vi "氨氮总磷质控流程.vi"(9 "总磷1":bool, 10 "氨氮1":bool, 11 "队列输入":refnum<queue>) -> (3 "布尔":bool)   [LabVIEW 2016, in "质控单元.lvlib"]
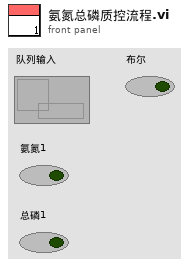
[diagram p1: front panel]
types:
  T1 = enum16{"待机", "启动氨氮水样", "氨氮测量中", "启动氨氮加标", "启动氨氮加标回收", "氨氮加标回收测量中", "启动总磷水样", "总磷水样测量中", "启动总磷加标", "启动总磷加标回收", "总磷加标回收测量中", "结束"}
  T2 = cluster{"站号":u16, "量程切换":enum32{"H", "L", "AUTO"}, "控制命令":enum16{"启动测量", "标样核查", "零点核查", "跨度核查", "空白测试", "平行样测试", "加标回收", "空白校准", "标样校准", "初始化（清洗）", "停止测试", "仪器重启", "校时", "模式设置", "测量间隔设置", "盲样测试"}, "模式设置":enum16{"待机", "连续模式", "周期模式", "定点模式", "受控模式", "手动模式"}, "测量间隔":u16}
  T3 = cluster{"时间标识":timestamp, "设备":string, "日志信息":string}
  T4 = cluster{"系统时间":timestamp, "工作状态":enum16{"空闲", "水样测试", "标样核查", "零点核查", "跨度核查", "空白测试", "平行样测试", "加标回收", "空白校准", "标样校准", "初始化（清洗）"}, "测量模式":enum16{"待机", "连续模式", "周期模式", "定点模式", "受控模式", "手动模式"}, "告警代码":enum16{"无告警", "缺试剂告警", "缺水样告警", "缺蒸馏水告警", "缺标液告警", "仪表漏液告警", "标定异常告警", "超量程告警", "加热异常", "低试剂预警", "超上限告警", "超下限告警", "仪表内部其他异常", "滴定异常告警", "电极异常告警", "量程切换告警", "参数设置告警", "PH电极电位异常", "电导率电极异常", "浊度光度异常", "溶解氧电极异常", "溶解氧光强异常", "温度异常告警", "PH异常告警", "溶解氧异常告警", "电导率异常告警", "浊度异常告警", "叶绿素异常告警", "藻密度异常告警", "蓝绿藻异常告警", "ORP异常告警", "氨氮异常告警", "清洁刷异常告警", "SD卡异常告警", "蓝牙异常告警", "Wifi异常告警", "流程异常告警"}, "故障代码":enum16{"无故障", "电机故障", "温度故障", "通讯故障", "滴定故障"}, "日志代码":u16, "软件版本":u16, "F0":sgl, "F1":sgl, "F2":sgl, "F3":sgl, "T":sgl, "H":sgl, "id":u16, "flowid":u16, "量程":u16}
  T5 = enum16{"空闲", "水样测试", "标样核查", "零点核查", "跨度核查", "空白测试", "平行样测试", "加标回收", "空白校准", "标样校准", "初始化（清洗）"}
  T6 = cluster{"因子编码":u32, "单位":u16, "标样参考值":sgl, "水样数据时间":timestamp, "水样实测值":sgl, "水样数据标识":string, "标样数据时间":timestamp, "标样实测值":sgl, "标样数据标识":string, "空白数据时间":timestamp, "空白实测值":sgl, "空白数据标识":string, "零点核查数据时间":timestamp, "零点核查实测值":sgl, "零点核查数据标识":string, "跨度核查数据时间":timestamp, "跨度核查实测值":sgl, "跨度核查数据标识":string, "加标回收数据时间":timestamp, "加标回收实测值":sgl, "加标回收数据标识":string, "平行样数据时间":timestamp, "平行样实测值":sgl, "平行样数据标识":string}
  T7 = cluster{"量程":dbl, "检出限":dbl, "加标前水样浓度":dbl, "加标后水样浓度":dbl, "加标水杯定容体积":dbl, "加标母液浓度":dbl, "加标体积":dbl, "加标回收率":dbl}
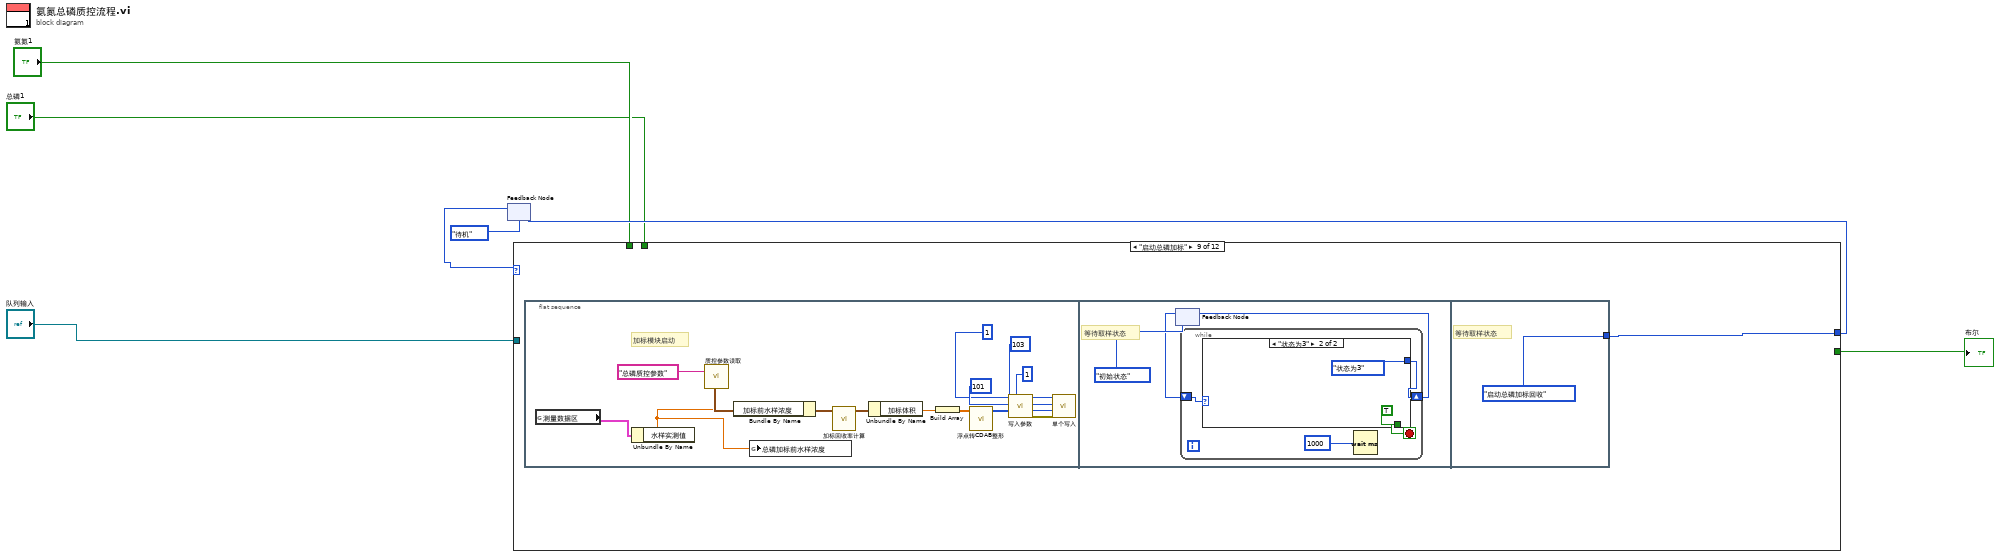
[diagram p0: block diagram]
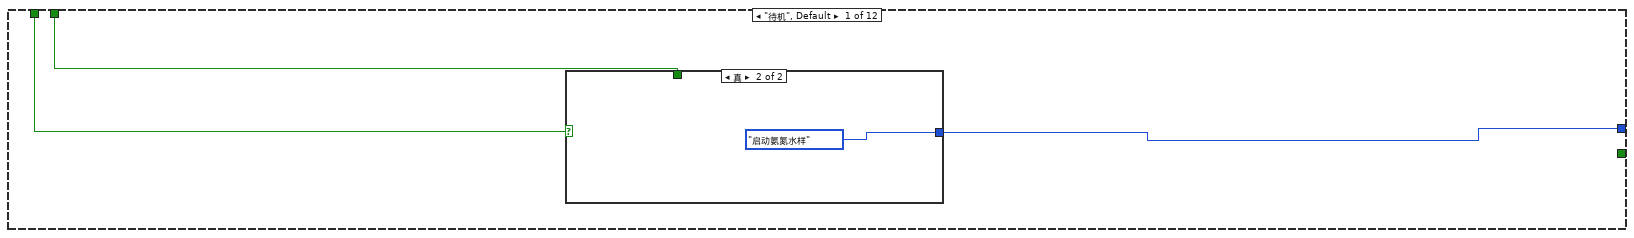
[diagram p2: hidden frame]
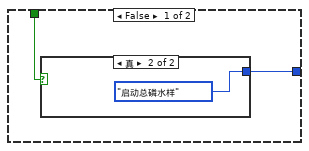
[diagram p3: hidden frame]
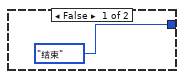
[diagram p4: hidden frame]
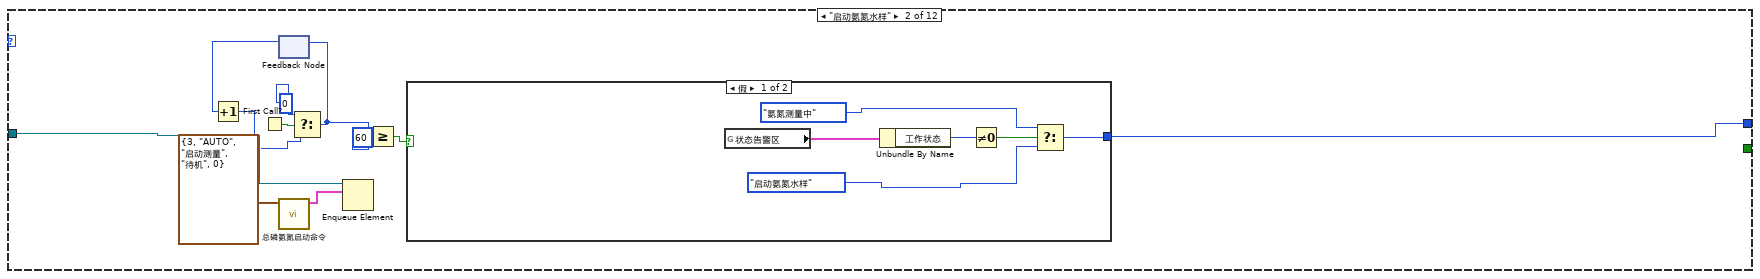
[diagram p5: hidden frame]
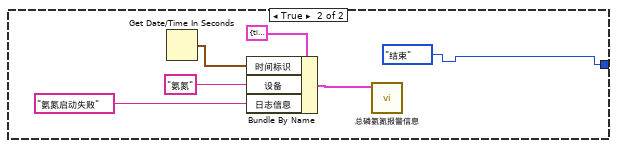
[diagram p6: hidden frame]
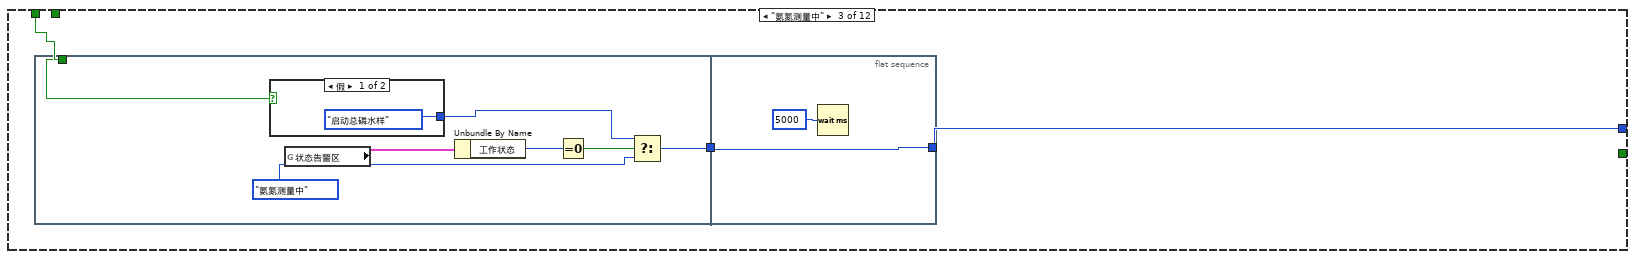
[diagram p7: hidden frame]
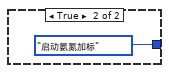
[diagram p8: hidden frame]
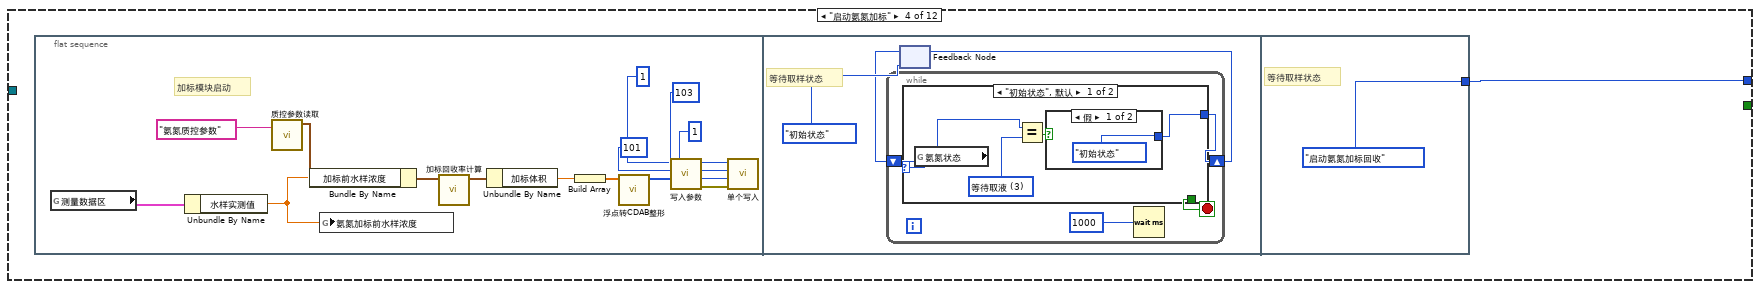
[diagram p9: hidden frame]
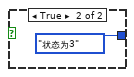
[diagram p10: hidden frame]
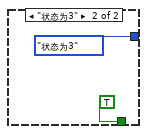
[diagram p11: hidden frame]
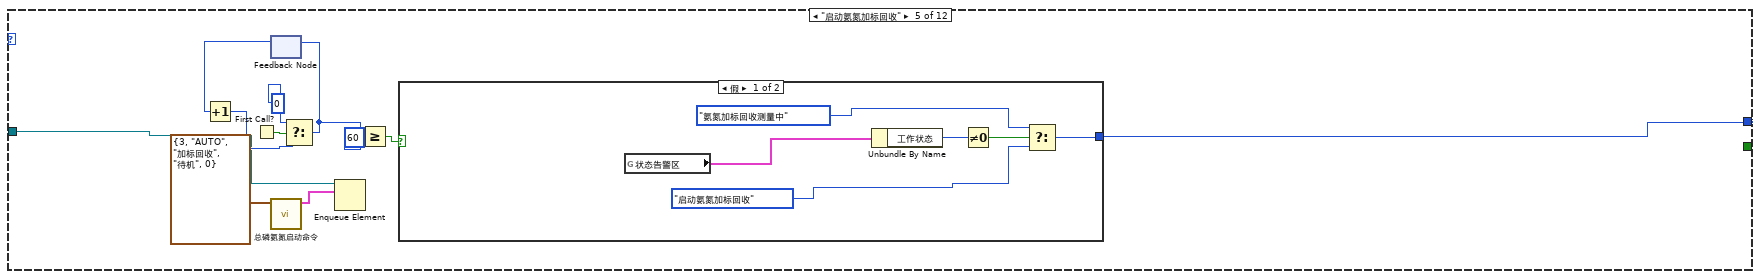
[diagram p12: hidden frame]
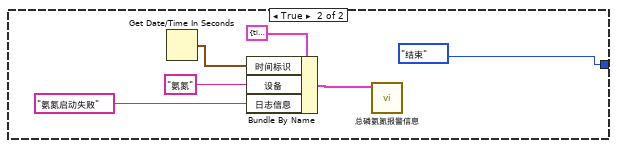
[diagram p13: hidden frame]
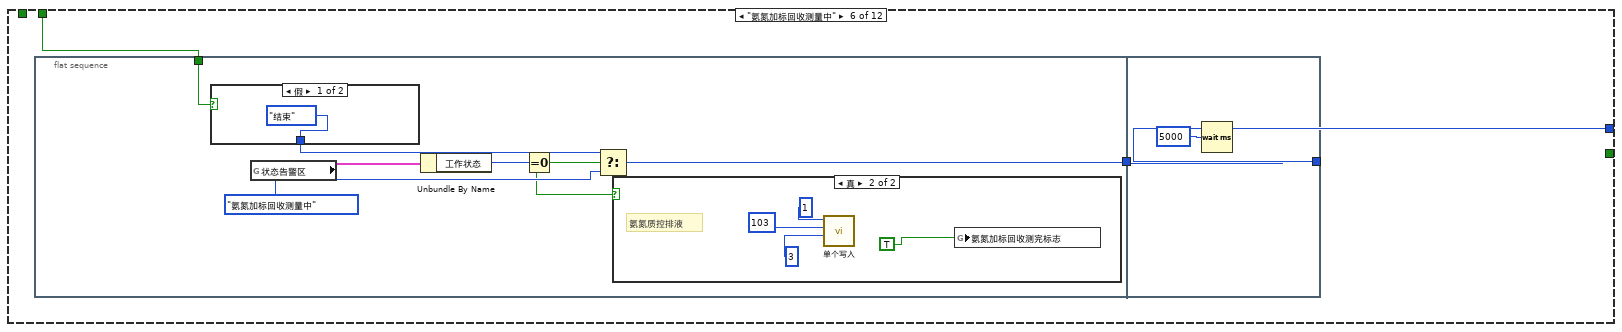
[diagram p14: hidden frame]
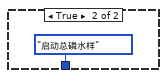
[diagram p15: hidden frame]
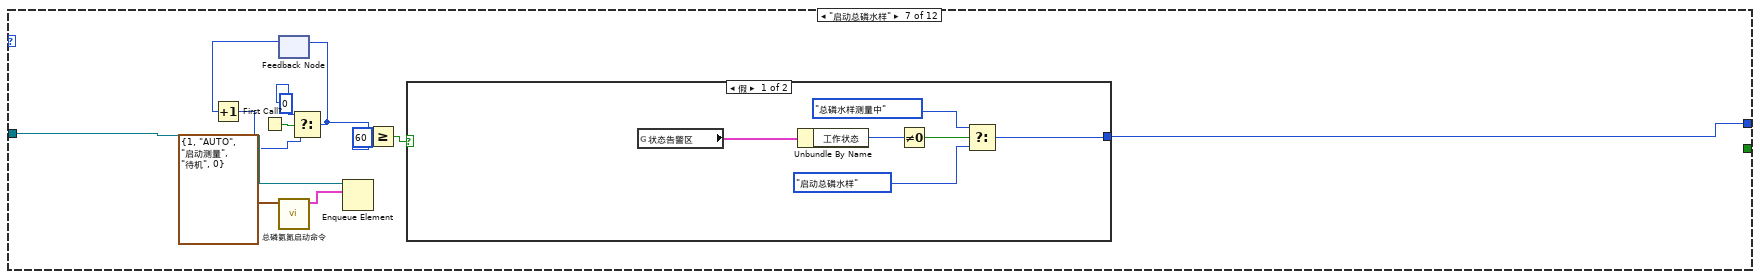
[diagram p17: hidden frame]
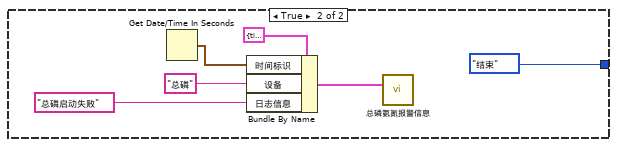
[diagram p18: hidden frame]
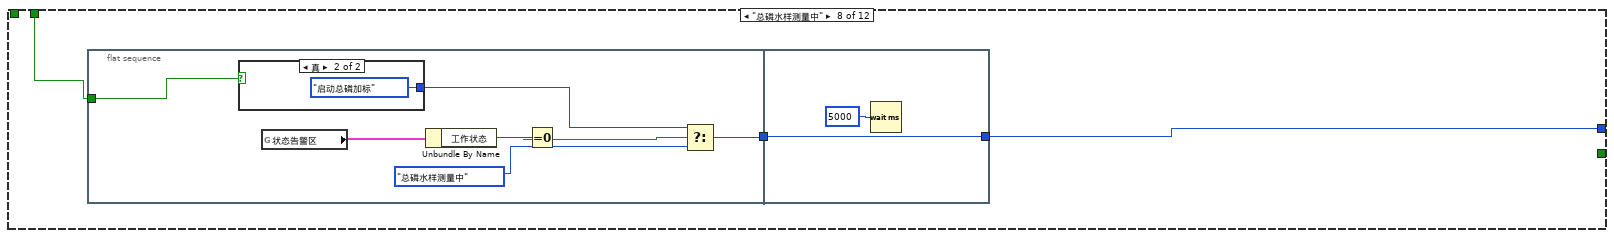
[diagram p19: hidden frame]
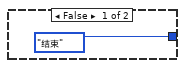
[diagram p20: hidden frame]
diagram:
  n1 = feedback #1(T1."待机") -> (w6:T1)
  n2 = case shown="\"启动总磷加标\"" w6 {
    tunnel: [w10 w25 w41 w53 w84 w108 w134 w150 w162 w193 w216 T1."结束"] -> w5
    tunnel: "队列输入" -> [_ w26 _ _ w85 _ w135 _ _ w194 _ _]
    tunnel: [_ _ _ _ _ _ _ _ _ _ _ TRUE] -> w2
    tunnel: "总磷1" -> [w8 _ _ _ _ w107 _ w148 _ _ _ _]
    tunnel: "氨氮1" -> [w9 _ w39 _ _ _ _ _ _ _ _ _]
    frame "待机", Default {
      n3 = case shown="真" w9 {
        tunnel: [w11 T1."启动氨氮水样"] -> w10
        tunnel: w8 -> [w12 _]
        frame False {
          n4 = case shown="真" w12 {
            tunnel: [T1."结束" T1."启动总磷水样"] -> w11
            frame False {
            }
            frame True {
            }
          }
        }
        frame True {
        }
      }
    }
    frame "启动氨氮水样" {
      n5 = First Call?() -> (First Call?: T/F=w23:bool)
      n6 = feedback #2() -> (w22:i32)  [unwired: 1 in]
      n7 = Increment(x=w22) -> (x+1=w21:i32)
      n8 = call "总磷氨氮启动命令.vi"("参数"=T2 {"站号"=3, "量程切换"=enum."AUTO", "控制命令"=enum."启动测量", "模式设置"=enum."待机", "测量间隔"=0}) -> ("启动命令"=w17:cluster{"命令":string, "data":variant})  [unwired: 10 in]
      n9 = Select(t=0, s=w23, f=w21) -> (s? t:f=w20:i32)
      n10 = feedback-in #2(w20) -> ()
      n11 = Enqueue Element(queue=w26, element=w17) -> ()  [unwired: 2 in, 3 out]
      n12 = Greater Or Equal?(x=w20, y=60) -> (x >= y?=w18:bool)
      n13 = case shown="假" w18 {
        tunnel: [w29 T1."结束"] -> w25
        frame False {
          n14 = global read "VAR总磷氨氮全局变量.vi" "状态告警区"() -> (w32:T4)
          n15 = Unbundle By Name(w32) -> ("工作状态"=w31:T5)
          n16 = Not Equal To 0?(x=w31) -> (x != 0?=w30:bool)
          n17 = Select(t=T1."氨氮测量中", s=w30, f=T1."启动氨氮水样") -> (s? t:f=w29:T1)
        }
        frame True {
          n18 = Get Date/Time In Seconds() -> (seconds since 1Jan1904=w38:timestamp)
          n19 = Bundle By Name(cluster=T3 {"时间标识"=timestamp(0 s since 1904-01-01), "设备"="", "日志信息"=""} ("data in"), "时间标识"=w38, "设备"="氨氮", "日志信息"="氨氮启动失败") -> (w34:T3)
          n20 = call "总磷氨氮报警信息.vi"("data in"=w34) -> ()  [unwired: 11 in]
        }
      }
    }
    frame "氨氮测量中" {
      n21 = flat-sequence {
        tunnel: [w46] -> w40
        tunnel: w39 -> [w42]
        tunnel: [w52] -> w41
        tunnel: w40 -> [w52]
        frame #0 {
          n22 = case shown="假" w42 {
            tunnel: [T1."启动总磷水样" T1."启动氨氮加标"] -> w43
            frame False {
            }
            frame True {
            }
          }
          n23 = global read "VAR总磷氨氮全局变量.vi" "状态告警区"() -> (w47:T4)
          n24 = Unbundle By Name(w47) -> ("工作状态"=w48:T5)
          n25 = Equal To 0?(x=w48) -> (x = 0?=w45:bool)
          n26 = Select(t=w43, s=w45, f=T1."氨氮测量中") -> (s? t:f=w46:T1)
        }
        frame #1 {
          n27 = Wait (ms)(milliseconds to wait=u32 5000 ("等待时间（毫秒）")) -> ()  [unwired: 1 out]
        }
      }
    }
    frame "启动氨氮加标" {
      n28 = flat-sequence {
        tunnel: [T1."启动氨氮加标回收"] -> w53
        frame #0 {
          w57 = u16 1 ("value")
          # "加标模块启动"
          n29 = global read "VAR总磷氨氮全局变量.vi" "测量数据区"() -> (w55:T6)
          n30 = Unbundle By Name(w55) -> ("水样实测值"=w54:sgl)
          n31 = call "质控参数读取.vi"("section"="氨氮质控参数") -> ("参数"=w65:T7)  [unwired: 9 in, 1 out]
          n32 = Bundle By Name(cluster=w65, "加标前水样浓度"=w54) -> (w66:T7)
          n33 = global write "水样浓度全局.vi" "氨氮加标前水样浓度"(w54) -> ()
          n34 = call "加标回收率计算.vi"("参数"=w66) -> ("参数 out"=w64:T7)  [unwired: 10 in]
          n35 = Unbundle By Name(w64) -> ("加标体积"=w56:dbl)
          n36 = Build Array(w56) -> (w63:dbl[])
          n37 = call "浮点转CDAB整形.vi"("浮点数"=w63) -> ("CDAB整形输出"=w58:u16[])  [unwired: 10 in]
          n38 = call "写入参数.vi"("values"=w58, "starting address"=u16 101, "Slave ID"=w57) -> ("error out"=w62:errorcluster)  [unwired: 8 in]
          n39 = call "单个写入.vi"("Error in"=w62, "value"=u16 1, "address"=u16 103, "Slave ID"=w57) -> ()  [unwired: 7 in, 1 out]
        }
        frame #1 {
          # "等待取样状态"
          n40 = feedback #3(enum16{"初始状态", "状态为3"}."初始状态") -> (w69:enum16{"初始状态", "状态为3"})
          n41 = while {
            shift-right: [w73] -> w68
            shift-left: w69 -> [w74]
            stop <- w72 stop-if-true
            n42 = case shown="\"初始状态\", 默认" w74 {
              tunnel: [w76 enum16{"初始状态", "状态为3"}."状态为3"] -> w73
              tunnel: [_ TRUE] -> w72
              frame "初始状态", Default {
                w75 = u16 3 items=["待机", "润洗", "进样", "等待取液", "排液"] ("氨氮状态")
                n43 = global read "氨氮加标回收状态全局变量.vi" "氨氮状态"() -> (w78:u16)
                n44 = Equal?(x=w78, y=w75) -> (x = y?=w77:bool)
                n45 = case shown="假" w77 {
                  tunnel: [enum16{"初始状态", "状态为3"}."初始状态" enum16{"初始状态", "状态为3"}."状态为3"] -> w76
                  frame False {
                  }
                  frame True {
                  }
                }
              }
              frame "状态为3" {
              }
            }
            n46 = Wait (ms)(milliseconds to wait=u32 1000 ("等待时间（毫秒）")) -> ()  [unwired: 1 out]
          }
          n47 = feedback-in #3(w68) -> ()
        }
        frame #2 {
          # "等待取样状态"
        }
      }
    }
    frame "启动氨氮加标回收" {
      n48 = First Call?() -> (First Call?: T/F=w93:bool)
      n49 = feedback #4() -> (w92:i32)  [unwired: 1 in]
      n50 = Increment(x=w92) -> (x+1=w91:i32)
      n51 = call "总磷氨氮启动命令.vi"("参数"=T2 {"站号"=3, "量程切换"=enum."AUTO", "控制命令"=enum."加标回收", "模式设置"=enum."待机", "测量间隔"=0}) -> ("启动命令"=w87:cluster{"命令":string, "data":variant})  [unwired: 10 in]
      n52 = Select(t=0, s=w93, f=w91) -> (s? t:f=w90:i32)
      n53 = feedback-in #4(w90) -> ()
      n54 = Enqueue Element(queue=w85, element=w87) -> ()  [unwired: 2 in, 3 out]
      n55 = Greater Or Equal?(x=w90, y=60) -> (x >= y?=w88:bool)
      n56 = case shown="假" w88 {
        tunnel: [w97 T1."结束"] -> w84
        frame False {
          n57 = global read "VAR总磷氨氮全局变量.vi" "状态告警区"() -> (w100:T4)
          n58 = Unbundle By Name(w100) -> ("工作状态"=w99:T5)
          n59 = Not Equal To 0?(x=w99) -> (x != 0?=w98:bool)
          n60 = Select(t=T1."氨氮加标回收测量中", s=w98, f=T1."启动氨氮加标回收") -> (s? t:f=w97:T1)
        }
        frame True {
          n61 = Get Date/Time In Seconds() -> (seconds since 1Jan1904=w106:timestamp)
          n62 = Bundle By Name(cluster=T3 {"时间标识"=timestamp(0 s since 1904-01-01), "设备"="", "日志信息"=""} ("data in"), "时间标识"=w106, "设备"="氨氮", "日志信息"="氨氮启动失败") -> (w102:T3)
          n63 = call "总磷氨氮报警信息.vi"("data in"=w102) -> ()  [unwired: 11 in]
        }
      }
    }
    frame "氨氮加标回收测量中" {
      n64 = flat-sequence {
        tunnel: [w114] -> w109
        tunnel: w107 -> [w110]
        tunnel: [w124] -> w108
        tunnel: w109 -> [w124]
        frame #0 {
          n65 = case shown="假" w110 {
            tunnel: [T1."结束" T1."启动总磷水样"] -> w112
            frame False {
            }
            frame True {
            }
          }
          n66 = global read "VAR总磷氨氮全局变量.vi" "状态告警区"() -> (w115:T4)
          n67 = Unbundle By Name(w115) -> ("工作状态"=w116:T5)
          n68 = Equal To 0?(x=w116) -> (x = 0?=w111:bool)
          n69 = Select(t=w112, s=w111, f=T1."氨氮加标回收测量中") -> (s? t:f=w114:T1)
          n70 = case shown="真" w111 {
            frame False {
            }
            frame True {
              # "氨氮质控排液"
              n71 = call "单个写入.vi"("value"=u16 3, "address"=u16 103, "Slave ID"=u8 1) -> ()  [unwired: 8 in, 1 out]
              n72 = global write "质控测完标志全局 1.vi" "氨氮加标回收测完标志"(TRUE) -> ()
            }
          }
        }
        frame #1 {
          n73 = Wait (ms)(milliseconds to wait=u32 5000 ("等待时间（毫秒）")) -> ()  [unwired: 1 out]
        }
      }
    }
    frame "启动总磷水样" {
      n74 = First Call?() -> (First Call?: T/F=w132:bool)
      n75 = feedback #5() -> (w131:i32)  [unwired: 1 in]
      n76 = Increment(x=w131) -> (x+1=w130:i32)
      n77 = call "总磷氨氮启动命令.vi"("参数"=T2 {"站号"=1, "量程切换"=enum."AUTO", "控制命令"=enum."启动测量", "模式设置"=enum."待机", "测量间隔"=0}) -> ("启动命令"=w126:cluster{"命令":string, "data":variant})  [unwired: 10 in]
      n78 = Select(t=0, s=w132, f=w130) -> (s? t:f=w129:i32)
      n79 = feedback-in #5(w129) -> ()
      n80 = Enqueue Element(queue=w135, element=w126) -> ()  [unwired: 2 in, 3 out]
      n81 = Greater Or Equal?(x=w129, y=60) -> (x >= y?=w127:bool)
      n82 = case shown="假" w127 {
        tunnel: [w138 T1."结束"] -> w134
        frame False {
          n83 = global read "VAR总磷氨氮全局变量.vi" "状态告警区"() -> (w139:T4)
          n84 = Unbundle By Name(w139) -> ("工作状态"=w140:T5)
          n85 = Not Equal To 0?(x=w140) -> (x != 0?=w141:bool)
          n86 = Select(t=T1."总磷水样测量中", s=w141, f=T1."启动总磷水样") -> (s? t:f=w138:T1)
        }
        frame True {
          n87 = Get Date/Time In Seconds() -> (seconds since 1Jan1904=w147:timestamp)
          n88 = Bundle By Name(cluster=T3 {"时间标识"=timestamp(0 s since 1904-01-01), "设备"="", "日志信息"=""} ("data in"), "时间标识"=w147, "设备"="总磷", "日志信息"="总磷启动失败") -> (w143:T3)
          n89 = call "总磷氨氮报警信息.vi"("data in"=w143) -> ()  [unwired: 11 in]
        }
      }
    }
    frame "总磷水样测量中" {
      n90 = flat-sequence {
        tunnel: [w155] -> w149
        tunnel: w148 -> [w151]
        tunnel: [w161] -> w150
        tunnel: w149 -> [w161]
        frame #0 {
          n91 = case shown="真" w151 {
            tunnel: [T1."结束" T1."启动总磷加标"] -> w153
            frame False {
            }
            frame True {
            }
          }
          n92 = global read "VAR总磷氨氮全局变量.vi" "状态告警区"() -> (w156:T4)
          n93 = Unbundle By Name(w156) -> ("工作状态"=w157:T5)
          n94 = Equal To 0?(x=w157) -> (x = 0?=w154:bool)
          n95 = Select(t=w153, s=w154, f=T1."总磷水样测量中") -> (s? t:f=w155:T1)
        }
        frame #1 {
          n96 = Wait (ms)(milliseconds to wait=u32 5000 ("等待时间（毫秒）")) -> ()  [unwired: 1 out]
        }
      }
    }
    frame "启动总磷加标" {
      n97 = flat-sequence {
        tunnel: [T1."启动总磷加标回收"] -> w162
        frame #0 {
          w167 = u16 1 ("value")
          # "加标模块启动"
          n98 = global read "VAR总磷氨氮全局变量.vi" "测量数据区"() -> (w165:T6)
          n99 = Unbundle By Name(w165) -> ("水样实测值"=w163:sgl)
          n100 = call "质控参数读取.vi"("section"="总磷质控参数") -> ("参数"=w164:T7)  [unwired: 9 in, 1 out]
          n101 = Bundle By Name(cluster=w164, "加标前水样浓度"=w163) -> (w175:T7)
          n102 = global write "水样浓度全局.vi" "总磷加标前水样浓度"(w163) -> ()
          n103 = call "加标回收率计算.vi"("参数"=w175) -> ("参数 out"=w174:T7)  [unwired: 10 in]
          n104 = Unbundle By Name(w174) -> ("加标体积"=w166:dbl)
          n105 = Build Array(w166) -> (w173:dbl[])
          n106 = call "浮点转CDAB整形.vi"("浮点数"=w173) -> ("CDAB整形输出"=w168:u16[])  [unwired: 10 in]
          n107 = call "写入参数.vi"("values"=w168, "starting address"=u16 101, "Slave ID"=w167) -> ("error out"=w172:errorcluster)  [unwired: 8 in]
          n108 = call "单个写入.vi"("Error in"=w172, "value"=u16 1, "address"=u16 103, "Slave ID"=w167) -> ()  [unwired: 7 in, 1 out]
        }
        frame #1 {
          # "等待取样状态"
          n109 = feedback #6(enum16{"初始状态", "状态为3"}."初始状态") -> (w178:enum16{"初始状态", "状态为3"})
          n110 = while {
            shift-right: [w182] -> w177
            shift-left: w178 -> [w183]
            stop <- w181 stop-if-true
            n111 = case shown="\"状态为3\"" w183 {
              tunnel: [w184 enum16{"初始状态", "状态为3"}."状态为3"] -> w182
              tunnel: [_ TRUE] -> w181
              frame "初始状态", Default {
                n112 = global read "氨氮加标回收状态全局变量.vi" "总磷状态"() -> (w186:u16)
                n113 = Equal?(x=w186, y=u16 3) -> (x = y?=w185:bool)
                n114 = case shown="真" w185 {
                  tunnel: [enum16{"初始状态", "状态为3"}."初始状态" enum16{"初始状态", "状态为3"}."状态为3"] -> w184
                  frame False {
                  }
                  frame True {
                  }
                }
              }
              frame "状态为3" {
              }
            }
            n115 = Wait (ms)(milliseconds to wait=u32 1000 ("等待时间（毫秒）")) -> ()  [unwired: 1 out]
          }
          n116 = feedback-in #6(w177) -> ()
        }
        frame #2 {
          # "等待取样状态"
        }
      }
    }
    frame "启动总磷加标回收" {
      n117 = First Call?() -> (First Call?: T/F=w202:bool)
      n118 = feedback #7() -> (w201:i32)  [unwired: 1 in]
      n119 = Increment(x=w201) -> (x+1=w200:i32)
      n120 = call "总磷氨氮启动命令.vi"("参数"=T2 {"站号"=1, "量程切换"=enum."AUTO", "控制命令"=enum."加标回收", "模式设置"=enum."待机", "测量间隔"=0}) -> ("启动命令"=w196:cluster{"命令":string, "data":variant})  [unwired: 10 in]
      n121 = Select(t=0, s=w202, f=w200) -> (s? t:f=w199:i32)
      n122 = feedback-in #7(w199) -> ()
      n123 = Enqueue Element(queue=w194, element=w196) -> ()  [unwired: 2 in, 3 out]
      n124 = Greater Or Equal?(x=w199, y=60) -> (x >= y?=w197:bool)
      n125 = case shown="假" w197 {
        tunnel: [w206 T1."结束"] -> w193
        frame False {
          n126 = global read "VAR总磷氨氮全局变量.vi" "状态告警区"() -> (w207:T4)
          n127 = Unbundle By Name(w207) -> ("工作状态"=w208:T5)
          n128 = Not Equal To 0?(x=w208) -> (x != 0?=w209:bool)
          n129 = Select(t=T1."总磷加标回收测量中", s=w209, f=T1."启动总磷加标回收") -> (s? t:f=w206:T1)
        }
        frame True {
          n130 = Get Date/Time In Seconds() -> (seconds since 1Jan1904=w215:timestamp)
          n131 = Bundle By Name(cluster=T3 {"时间标识"=timestamp(0 s since 1904-01-01), "设备"="", "日志信息"=""} ("data in"), "时间标识"=w215, "设备"="总磷", "日志信息"="总磷启动失败") -> (w211:T3)
          n132 = call "总磷氨氮报警信息.vi"("data in"=w211) -> ()  [unwired: 11 in]
        }
      }
    }
    frame "总磷加标回收测量中" {
      n133 = flat-sequence {
        tunnel: [w221] -> w217
        tunnel: [w229] -> w216
        tunnel: w217 -> [w229]
        frame #0 {
          n134 = global read "VAR总磷氨氮全局变量.vi" "状态告警区"() -> (w222:T4)
          n135 = Unbundle By Name(w222) -> ("工作状态"=w223:T5)
          n136 = Equal To 0?(x=w223) -> (x = 0?=w218:bool)
          n137 = Select(t=T1."结束", s=w218, f=T1."总磷加标回收测量中") -> (s? t:f=w221:T1)
          n138 = case shown="真" w218 {
            frame False {
            }
            frame True {
              # "总磷质控排液"
              n139 = global write "质控测完标志全局 1.vi" "氨氮总磷加标回收测完标志"(TRUE) -> ()
              n140 = call "单个写入.vi"("value"=u16 3, "address"=u16 103, "Slave ID"=u8 1) -> ()  [unwired: 8 in, 1 out]
            }
          }
        }
        frame #1 {
          n141 = Wait (ms)(milliseconds to wait=u32 5000 ("等待时间（毫秒）")) -> ()  [unwired: 1 out]
        }
      }
    }
    frame "结束" {
    }
  }
  "布尔" <- w2
  n142 = feedback-in #1(w5) -> ()
